vi "Get_Window_Saved.vi"(1 "VI Path":path) -> (0 "Saved":bool)   [LabVIEW 2011]
doc: "This VI returns true if the VI given by the \"VI Path\" parameter does not contain unsaved changes, otherwise it returns false."
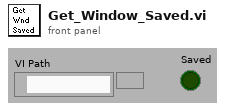
[diagram p1: front panel]
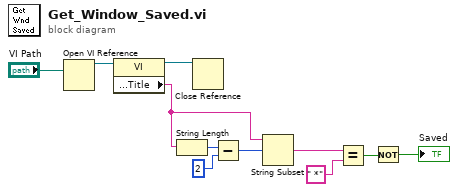
[diagram p0: block diagram]
diagram:
  n1 = Open VI Reference(vi path="VI Path") -> (vi reference=w11:refnum<vi>)  [unwired: 2 in, 4 out]
  n2 = property class="VI"(reference=w11) -> (reference out=w9:refnum<vi>, "Front Panel.Title"=w8:string)  [unwired: 1 in, 1 out]
  n3 = String Length(string=w8) -> (length=w7:i32)
  n4 = Close Reference(reference=w9) -> ()  [unwired: 1 in, 1 out]
  n5 = Subtract(x=w7, y=2) -> (x-y=w5:i32)
  n6 = String Subset(string=w8, offset (0)=w5) -> (substring=w4:string)  [unwired: 1 out]
  n7 = Equal?(x=w4, y=" *") -> (x = y?=w2:bool)
  n8 = Not(x=w2) -> (.not. x?=→"Saved":bool)
